vi "Multi Accelerometer Example.vi"() -> ()   [LabVIEW 2012, in "Phidget Common.lvlib"]
uses:
  <instrlib>/Phidgets/Phidget Common/Phidget Common.lvlib
  <instrlib>/Phidgets/Phidget Accelerometer/Public/AccelerometerClose.vi
  <instrlib>/Phidgets/Phidget Accelerometer/Public/AccelerometerStart.vi
  <instrlib>/Phidgets/Phidget Accelerometer/Phidget Accelerometer.lvlib
panel:
  out "Serial Number 2":i32
  out "Serial Number":i32
  out "error out 2":errorcluster
  in  "error in (no error) 2":errorcluster
  in  "Device Info 2":T1={"Serial Number"=-1, "Channel"=0, "Port"=0}
  out "Attached? 2":bool
  out "Accel Data 2":dbl[](array[numeric]) format="%.5f"
  out "error out":errorcluster
  in  "error in (no error)":errorcluster
  in  "Device Info":T1={"Serial Number"=-1, "Channel"=0, "Port"=0}
  out "Attached?":bool
  out "Accel Data":dbl[](array[numeric]) format="%.5f"
  # "With Multiple Devices, it is advised to specify\nthe serial number and channel of each device\nto identify them in operation."
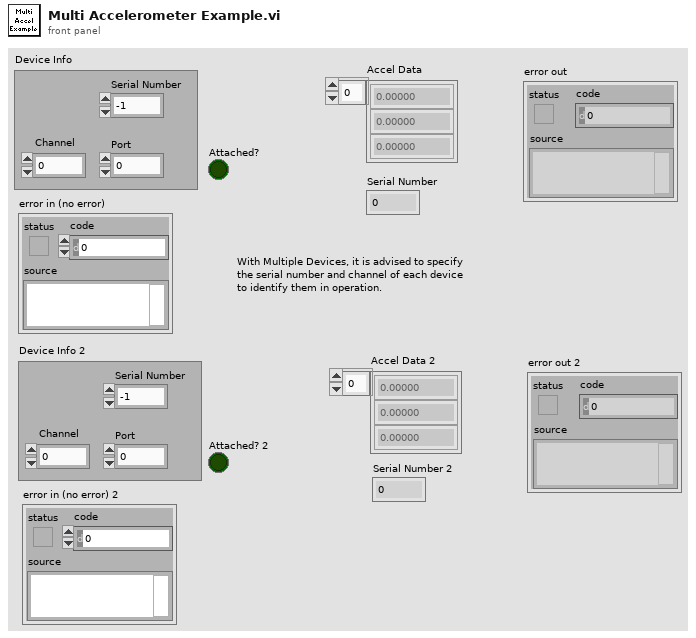
[diagram p1: front panel]
types:
  T1 = cluster{"Serial Number":i32, "Channel":i32, "Port":i32}
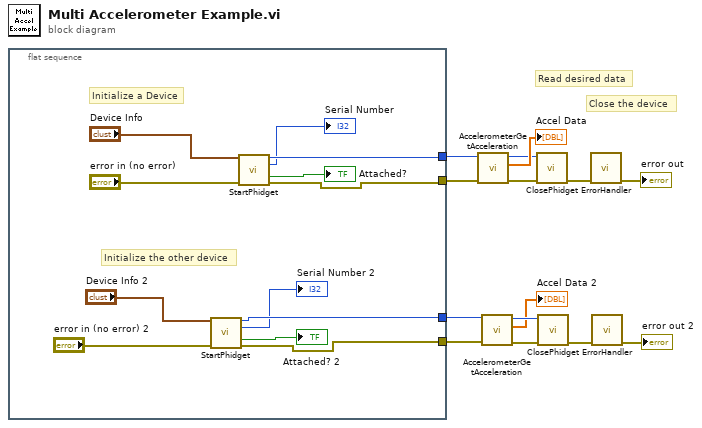
[diagram p0: block diagram]
diagram:
  # "Close the device"
  # "Read desired data"
  n1 = flat-sequence {
    tunnel: [w26] -> w14
    tunnel: [w25] -> w13
    tunnel: [w21] -> w10
    tunnel: [w20] -> w9
    frame #0 {
      # "Initialize the other device"
      # "Initialize a Device"
      n2 = call-poly <instrlib>:"StartPhidget.vi"("Device Info"="Device Info 2", "error in (no error)"="error in (no error) 2") -> ("Phidget ID"=w21:u64, "Serial Number Return"=→"Serial Number 2":i32, "Attached?"=→"Attached? 2":bool, "error out"=w20:errorcluster)  [unwired: 10 in]
      n3 = call-poly <instrlib>:"StartPhidget.vi"("Device Info"="Device Info", "error in (no error)"="error in (no error)") -> ("Phidget ID"=w26:u64, "Serial Number Return"=→"Serial Number":i32, "Attached?"=→"Attached?":bool, "error out"=w25:errorcluster)  [unwired: 10 in]
    }
  }
  n4 = call <instrlib>:"AccelerometerGetAcceleration.vi"("error in (no error)"=w13, "Device In"=w14) -> ("error out"=w4:errorcluster, "Acceleration"=→"Accel Data":dbl[], "Device Out"=w5:u64)  [unwired: 6 in]
  n5 = call <instrlib>:"AccelerometerGetAcceleration.vi"("error in (no error)"=w9, "Device In"=w10) -> ("error out"=w2:errorcluster, "Acceleration"=→"Accel Data 2":dbl[], "Device Out"=w3:u64)  [unwired: 6 in]
  n6 = call-poly <instrlib>:"ClosePhidget.vi"("error in"=w4, "Device In"=w5) -> ("error out"=w11:errorcluster)  [unwired: 9 in]
  n7 = call-poly <instrlib>:"ClosePhidget.vi"("error in"=w2, "Device In"=w3) -> ("error out"=w7:errorcluster)  [unwired: 9 in]
  n8 = call <instrlib>:"ErrorHandler.vi"("error in"=w11) -> ("error out"=→"error out":errorcluster)  [unwired: 9 in, 1 out]
  n9 = call <instrlib>:"ErrorHandler.vi"("error in"=w7) -> ("error out"=→"error out 2":errorcluster)  [unwired: 9 in, 1 out]
